vi "Configure Magnivu Enabled.vi"(8 "error in (no error)":errorcluster, 10 "Enable Magnivu (T: Enable)":bool=TRUE, 11 "VISA resource name":refnum<visa-resource-name>) -> (0 "error out":errorcluster, 3 "VISA resource name out":refnum<visa-resource-name>)   [LabVIEW 2016, in "Tektronix DPO MSO 2000 4000 Series.lvlib"]
doc: "Enables the MagniVu acquisition capability of the device to zoom into areas of interest on the waveform.\n\n<B>Note:</B> This VI is only valid for MSO 3000 and MSO 4000 models."
uses:
  Tektronix DPO MSO 2000 4000 Series.lvlib
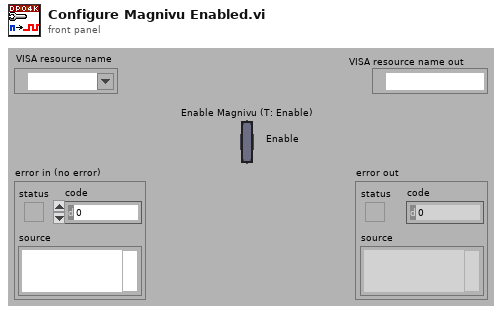
[diagram p1: front panel]
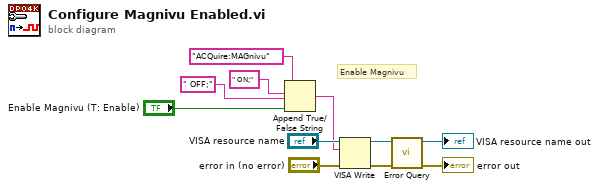
[diagram p0: block diagram]
diagram:
  # "Enable Magnivu"
  n1 = Append True/False String(1:"Enable Magnivu (T: Enable)", 2:" OFF;" ("false string"), 3:" ON;" ("true string"), 4:"ACQuire:MAGnivu" ("string (\"\")")) -> (0:w5:string)
  n2 = VISA Write(VISA resource name="VISA resource name", write buffer=w5, error in (no error)="error in (no error)") -> (VISA resource name out=w4:refnum<visa-resource-name>, error out=w3:errorcluster)  [unwired: 1 out]
  n3 = call "Error Query.vi"("error in (no error)"=w3, "VISA resource name"=w4) -> ("error out"=→"error out":errorcluster, "VISA resource name out"=→"VISA resource name out":refnum<visa-resource-name>)  [unwired: 6 in, 2 out]
